vi "Image Principle Measurements.vi"() -> ()   [LabVIEW 2016]
uses:
  <vilib>/userdefined/High Color/IMAQdx.ctl
  <vilib>/Utility/error.llb/DialogType.ctl
  <vilib>/vision/driver/NI_Vision_Acquisition_Software.lvlib
panel:
  in  "Pixel Measurement of the Standard":dbl=109.97 format="%#_13g"
  in  "Dimension of Standard in mm":dbl=2.0 format="%#_13g"
  in  "File Path for saving measurements":path
  out "Height Change in Pixels":dbl
  in  "File Path of Calibrated Image":path=path "C:/Users/user/Desktop/Studienarbeit Image Processing/Project File/Images/Calibration/Calibration_Target  Grid Distortion_Dot Dia_1mm/Template_Calibrated Image_Exposure_950.png"
  in  "Select the Pin to be measured":enum16{"1", "2", "3", "4", "5"}(ring)
  out "Pin Height in microns":dbl
  out "Pixel Size Coefficient":dbl
  out "Calibrated Image":T1(plugin-control)
  out "Image from Camera":T1(plugin-control)
  out "Error out at Process end":errorcluster
  in  "Stop Loop":bool
  in  "Image Acquistion Source":T2
  in  "Error in at IMAQ Create":errorcluster
  out "Error code out":i32 format="%0.0f"
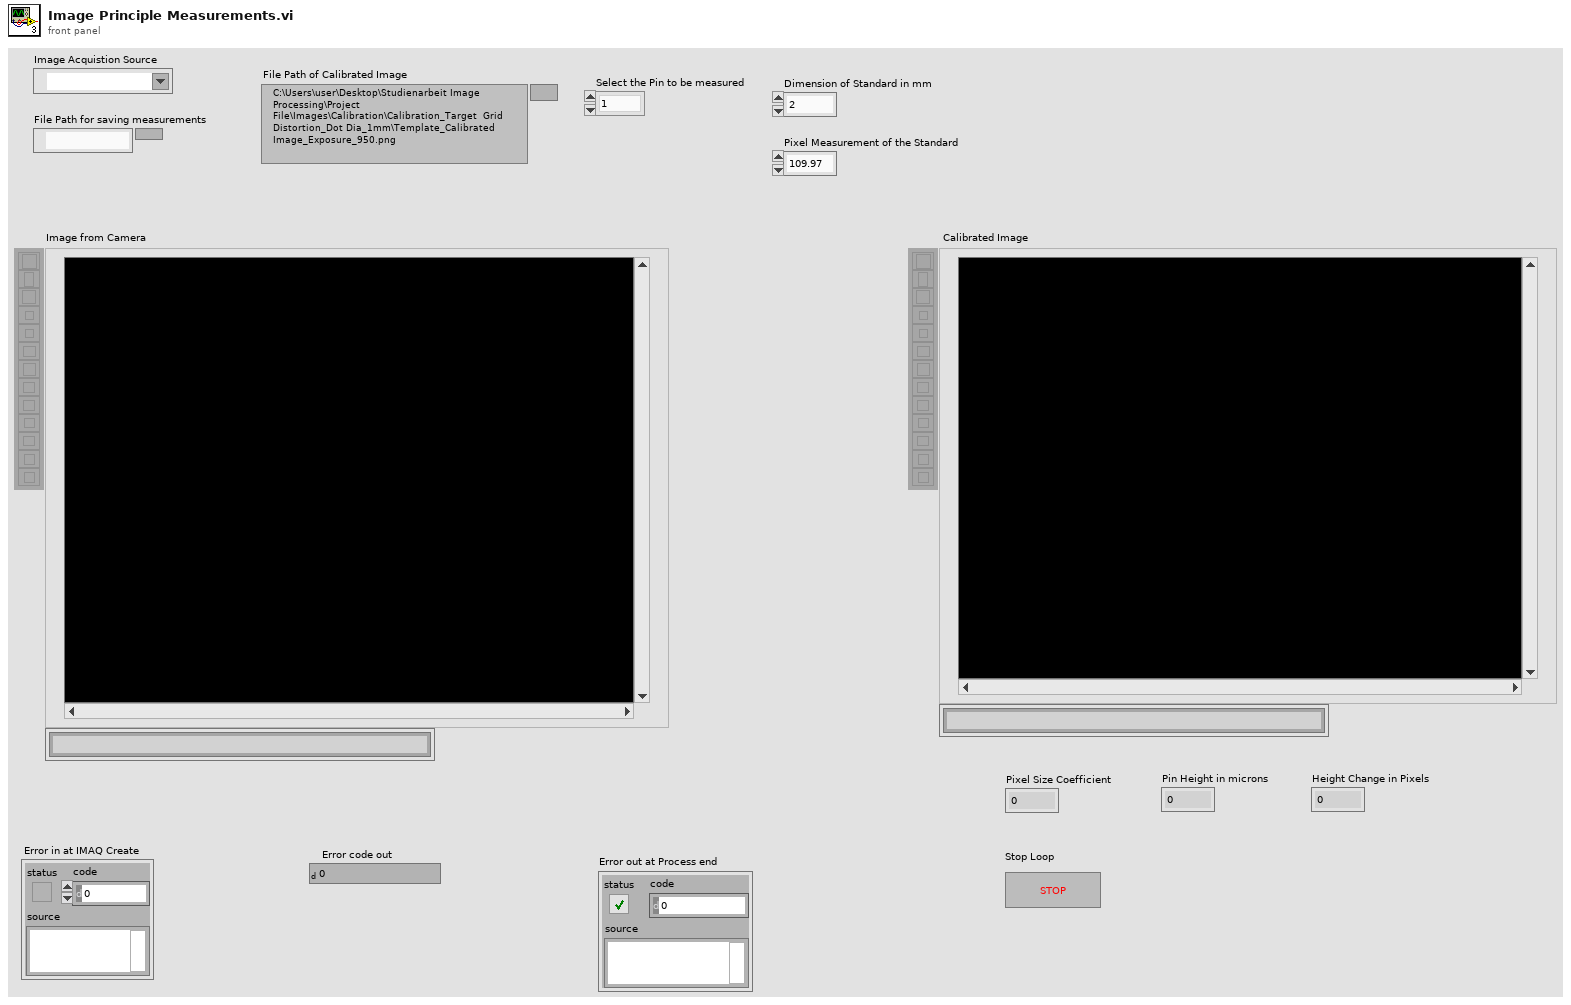
[diagram p1: front panel]
types:
  T1 = typedef "IMAQ Image.ctl" = refnum<image>
  T2 = typedef "IMAQdx.ctl" = refnum<k21>
  T3 = typedef "DialogType.ctl" = u16
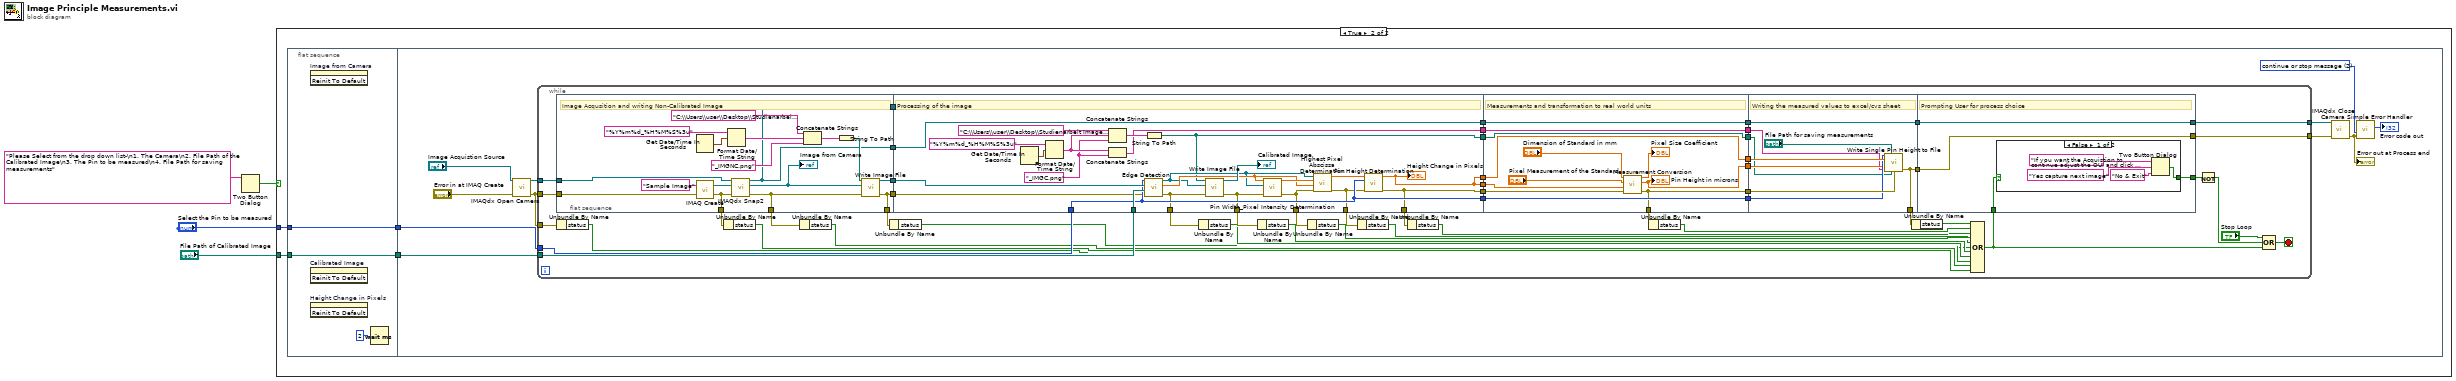
[diagram p0: block diagram]
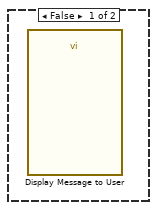
[diagram p2: hidden frame]
diagram:
  n1 = Two Button Dialog(message="Please Select from the drop down list-\n1. The Camera\n2. File Path of the Calibrated Image\n3. The Pin to be measured\n4. File Path for saving measurements") -> (T button?=w4:bool)  [unwired: 2 in]
  n2 = case shown="True" w4 {
    tunnel: "Select the Pin to be measured" -> [_ w8]
    tunnel: "File Path of Calibrated Image" -> [_ w6]
    frame False {
      n3 = call "Display Message to User"() -> ()  [unwired: 10 in, 2 out]
    }
    frame True {
      n4 = flat-sequence {
        tunnel: w8 -> [w10]
        tunnel: [w10] -> w7
        tunnel: w6 -> [w9]
        tunnel: [w9] -> w5
        tunnel: w7 -> [w16]
        tunnel: w5 -> [w17]
        frame #0 {
          n5 = invoke on="Image from Camera" class="ImageControl" method="Reinit To Default"() -> ()  [unwired: 3 in, 3 out]
          n6 = invoke on="Calibrated Image" class="ImageControl" method="Reinit To Default"() -> ()  [unwired: 3 in, 3 out]
          n7 = invoke on="Height Change in Pixels" class="DigNum (strict)" method="Reinit To Default"() -> ()  [unwired: 3 in, 3 out]
          n8 = Wait (ms)(milliseconds to wait=u32 2) -> ()  [unwired: 1 out]
        }
        frame #1 {
          w19 = T3 2 items=["no dialog", "OK message", "continue or stop message", "OK message + warnings", "continue/stop + warnings"] ("type of dialog (OK msg:1)")
          n9 = call <vilib>:"IMAQdx Open Camera.vi"("error in"="Error in at IMAQ Create", "Session In"="Image Acquistion Source") -> ("error out"=w13:errorcluster, "Session Out"=w18:T2)  [unwired: 8 in]
          n10 = while {
            tunnel: w13 -> [w75]
            tunnel: w18 -> [w74]
            tunnel: w17 -> [w69]
            tunnel: w16 -> [w68]
            tunnel: [w61] -> w15
            tunnel: [w52] -> w14
            tunnel: w13 -> [w44]
            stop <- w27 stop-if-true
            n11 = flat-sequence {
              tunnel: w75 -> [w92]
              tunnel: w74 -> [w91]
              tunnel: [w79] -> w73
              tunnel: [w78] -> w72
              tunnel: [w87] -> w71
              tunnel: [w79] -> w65
              tunnel: [w78] -> w47
              tunnel: [w77] -> w46
              tunnel: [w76] -> w45
              tunnel: w73 -> [_]
              tunnel: w72 -> [w98]
              tunnel: w71 -> [w109]
              tunnel: [w112] -> w70
              tunnel: w69 -> [w108]
              tunnel: w68 -> [w100]
              tunnel: [w99] -> w67
              tunnel: [w101] -> w66
              tunnel: w65 -> [w102]
              tunnel: [w102] -> w64
              tunnel: [w101] -> w57
              tunnel: [w100] -> w54
              tunnel: [w99] -> w49
              tunnel: [w97] -> w48
              tunnel: [w96] -> w43
              tunnel: [w95] -> w42
              tunnel: [w94] -> w41
              tunnel: [w93] -> w23
              tunnel: w70 -> [w118]
              tunnel: w67 -> [w127]
              tunnel: w66 -> [w126]
              tunnel: w64 -> [w123]
              tunnel: [w123] -> w63
              tunnel: [w119] -> w60
              tunnel: [w122] -> w58
              tunnel: w57 -> [w122]
              tunnel: [w121] -> w56
              tunnel: [w120] -> w55
              tunnel: w54 -> [w120]
              tunnel: [w119] -> w50
              tunnel: [w118] -> w53
              tunnel: [w117] -> w24
              tunnel: w23 -> [w117]
              tunnel: w63 -> [w137]
              tunnel: [w137] -> w62
              tunnel: w60 -> [w135]
              tunnel: [w136] -> w59
              tunnel: w58 -> [w133]
              tunnel: w56 -> [w131]
              tunnel: w55 -> [w132]
              tunnel: w53 -> [w130]
              tunnel: [w136] -> w51
              tunnel: w24 -> [w129]
              tunnel: w62 -> [w141]
              tunnel: [w141] -> w61
              tunnel: w59 -> [w140]
              tunnel: [w140] -> w52
              tunnel: w26 -> [w139]
              tunnel: [w138] -> w25
              frame #0 {
                # "Image Acqusition and writing Non-Calibrated Image"
                n12 = Get Date/Time In Seconds() -> (seconds since 1Jan1904=w82:timestamp)
                n13 = call "IMAQ Create"("Image Name"="Sample Image", "error in (no error)"=w92) -> ("New Image"=w90:T1, "error out"=w76:errorcluster)  [unwired: 3 in]
                n14 = Format Date/Time String(time format string (%c)="%Y%m%d_%H%M%S%3u", seconds (now)=w82) -> (date/time string=w85:string)  [unwired: 1 in]
                n15 = call <vilib>:"IMAQdx Snap2.vi"("error in"=w76, "Image In"=w90, "Session In"=w91) -> ("error out"=w77:errorcluster, "Image Out"=w88:T1, "Session Out"=w79:T2)  [unwired: 6 in]
                "Image from Camera" <- w88
                n16 = Concatenate Strings("C:\\Users\\user\\Desktop\\Studienarbeit Image Processing\\Project File\\Images\\Captured Images\\Images Non-Calibrated\\" ("string"), w85, "_IMGNC.png" ("string")) -> (w86:string)
                n17 = String To Path(string=w86) -> (path=w80:path)
                n18 = call "Write Image File.vi"("Error in at file creation"=w77, "Image to write"=w88, "File path for writing the file"=w80) -> ("Error out at image file writing"=w78:errorcluster, "Image Out after file writing"=w87:T1)  [unwired: 7 in]
              }
              frame #1 {
                w110 = "_IMGC.png" ("string")
                # "Processing of the image"
                n19 = Get Date/Time In Seconds() -> (seconds since 1Jan1904=w115:timestamp)
                n20 = Format Date/Time String(time format string (%c)="%Y%m%d_%H%M%S%3u", seconds (now)=w115) -> (date/time string=w111:string)  [unwired: 1 in]
                n21 = Concatenate Strings("C:\\Users\\user\\Desktop\\Studienarbeit Image Processing\\Project File\\Images\\Captured Images\\Images Calibrated with Vision Info\\" ("string"), w111, w110) -> (w113:string)
                n22 = Concatenate Strings(w111, w110) -> (w112:string)
                n23 = String To Path(string=w113) -> (path=w93:path)
                n24 = call "Edge Detection.vi"("error in (no error)"=w98, "File Path of Calibrated Image"=w108, "Image From Camera"=w109, "Select the Pin to be measured"=w100) -> ("error out"=w94:errorcluster, "Pixel Column of the edge"=w105:sgl, "Image"=w104:T1)  [unwired: 5 in]
                n25 = call "Write Image File.vi"("Error in at file creation"=w94, "Image to write"=w104, "File path for writing the file"=w93) -> ("Error out at image file writing"=w95:errorcluster, "Image Out after file writing"=→"Calibrated Image":T1)  [unwired: 7 in]
                n26 = call "Pin Width_Pixel Intensity Determination.vi"("error in"=w95, "Image"=w104, "Column Number from Edge Detection"=w105) -> ("error out"=w96:errorcluster, "Number of Dark Pixels from the edge"=w106:dbl)  [unwired: 7 in]
                n27 = call "Highest Pixel Abscissa Determination.vi"("error in"=w96, "Column Number from Edge Detection VI"=w105, "Pin Width from Pixel Intensity Determination VI"=w106, "Image"=w104) -> ("error out"=w97:errorcluster, "Pixel Value - Maximum Gradient occurs"=w103:dbl)  [unwired: 6 in]
                n28 = call "Pin Height Determination.vi"("Error In"=w97, "Pin number from Edge detection"=w100, "Pixel Value of Pin from Highest Pixel Abscissa Determination VI"=w103) -> ("Error Out"=w99:errorcluster, "Height in Pixels"=w101:dbl)  [unwired: 7 in]
                "Height Change in Pixels" <- w101
              }
              frame #2 {
                # "Measurements and transformation to real world units"
                n29 = call "Measurement Conversion.vi"("error in (no error)"=w127, "Pin height in pixels"=w126, "Pixel Measurement at Calibration"="Pixel Measurement of the Standard", "Dimension of Standard in mm"="Dimension of Standard in mm") -> ("error out"=w119:errorcluster, "Pin Measurement in microns"=w121:dbl, "Pixel Size Coefficient"=→"Pixel Size Coefficient":dbl)  [unwired: 5 in]
                "Pin Height in microns" <- w121
              }
              frame #3 {
                # "Writing the measured values to excel/cvs sheet"
                n30 = call "Write Single Pin Height to File.vi"("Pin Number"=w132, "File Path for saving measurements"="File Path for saving measurements", "Pin Height (Pixels)"=w133, "Pin Height (microns)"=w131, "Image Name"=w130, "Image File Destination"=w129, "Error at file writing"=w135) -> ("Error out at file writing"=w136:errorcluster)  [unwired: 7 in, 1 out]
              }
              frame #4 {
                # "Prompting User for process choice"
                n31 = case shown="False" w139 {
                  selector: w139 -> [_ w146]
                  tunnel: [w142 w146] -> w138
                  frame False {
                    n32 = Two Button Dialog(message="If you want the Acquistion to continue adjust the OUI and click on Yes", 1:"No & Exit" ("F button name (\"Cancel\")"), 2:"Yes capture next image" ("T button name (\"OK\")")) -> (T button?=w142:bool)
                  }
                  frame True {
                  }
                }
              }
            }
            n33 = Unbundle By Name(w44) -> ("status"=w30:bool)
            n34 = Unbundle By Name(w45) -> ("status"=w31:bool)
            n35 = Unbundle By Name(w46) -> ("status"=w32:bool)
            n36 = Unbundle By Name(w47) -> ("status"=w33:bool)
            n37 = Unbundle By Name(w41) -> ("status"=w34:bool)
            n38 = Unbundle By Name(w42) -> ("status"=w35:bool)
            n39 = Unbundle By Name(w43) -> ("status"=w37:bool)
            n40 = Unbundle By Name(w48) -> ("status"=w36:bool)
            n41 = Unbundle By Name(w49) -> ("status"=w38:bool)
            n42 = Unbundle By Name(w50) -> ("status"=w39:bool)
            n43 = Unbundle By Name(w51) -> ("status"=w40:bool)
            n44 = Compound Arithmetic op=OR(w40, w39, w38, w37, w36, w30, w35, w34, w33, w32, w31) -> (w26:bool)
            n45 = Not(x=w25) -> (.not. x?=w28:bool)
            n46 = Compound Arithmetic op=OR("Stop Loop", w28, w26) -> (w27:bool)
          }
          n47 = call <vilib>:"IMAQdx Close Camera.vi"("error in"=w14, "Session In"=w15) -> ("error out"=w12:errorcluster)  [unwired: 9 in]
          "Error out at Process end" <- w12
          n48 = call <vilib>:"Simple Error Handler.vi"("type of dialog (OK msg:1)"=w19, "error in (no error)"=w12) -> ("code out"=→"Error code out":i32)  [unwired: 3 in, 4 out]
        }
      }
    }
  }
